vi "Autonomous Independent.vi"   [LabVIEW 2019]
doc: "This VI is called when autonomous begins, and will automatically be terminated when autonomous ends. You can carry out timed or sensor driven robot movement independently without needing to return to the caller."
uses:
  <vilib>/Rock Robotics/WPI/Utilities/WPI_GetSetVariantRefNum.vi
  <vilib>/Rock Robotics/Network Tables/NT Read String.vi
  <vilib>/Rock Robotics/Network Tables/NT Write Numeric Array.vi
  Robot Global Data.vi
panel:
  # "Be sure to right-click and choose Data Operations>>Make Current Value default if you want to save the array values with the VI"
types:
  T1 = typedef "WPI_JoystickDevRef.ctl" = cluster{"Device":T2}
  T2 = typedef "WPI_JoystickDeviceEnum.ctl" = enum16{"USB 0", "USB 1", "USB 2", "USB 3", "USB 4", "USB 5"}
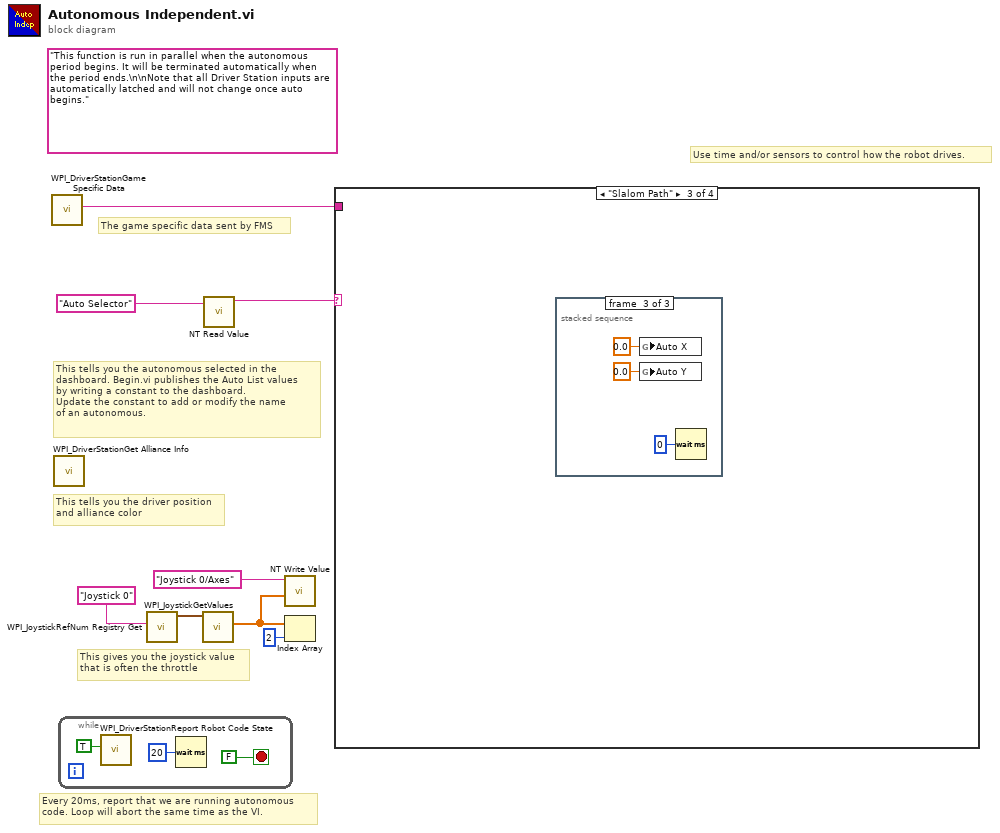
[diagram p0: block diagram]
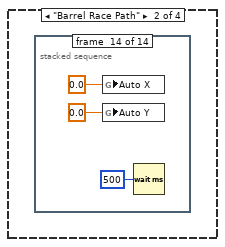
[diagram p3: hidden frame]
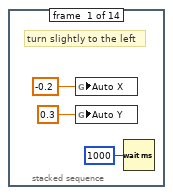
[diagram p4: hidden frame]
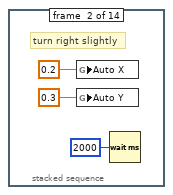
[diagram p5: hidden frame]
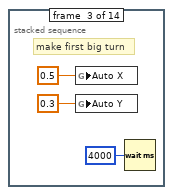
[diagram p6: hidden frame]
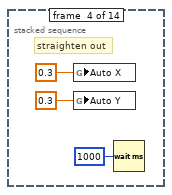
[diagram p7: hidden frame]
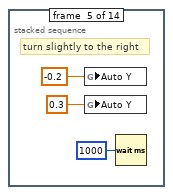
[diagram p8: hidden frame]
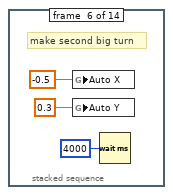
[diagram p9: hidden frame]
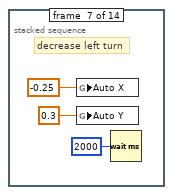
[diagram p10: hidden frame]
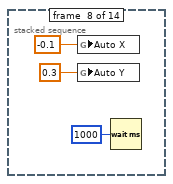
[diagram p11: hidden frame]
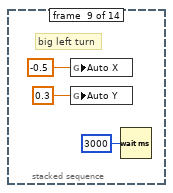
[diagram p12: hidden frame]
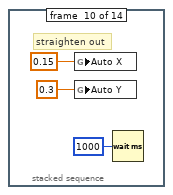
[diagram p13: hidden frame]
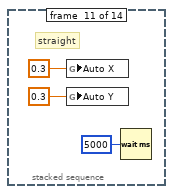
[diagram p14: hidden frame]
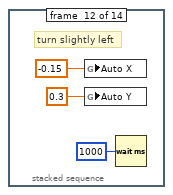
[diagram p15: hidden frame]
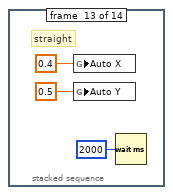
[diagram p16: hidden frame]
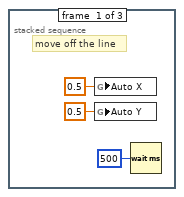
[diagram p17: hidden frame]
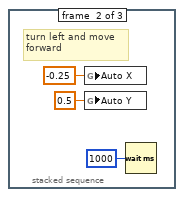
[diagram p18: hidden frame]
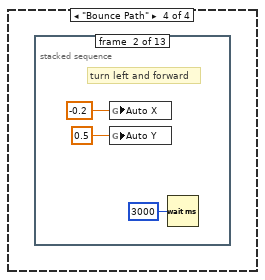
[diagram p19: hidden frame]
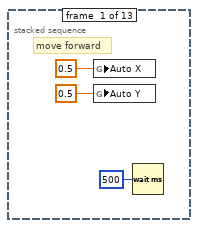
[diagram p20: hidden frame]
diagram:
  (unwired) "This function is run in parallel when the autonomous period begins. It will be terminated automatically when the period ends.\n\nNote that all Driver Station inputs are automatically latched and will not change once auto begins."
  # "The game specific data sent by FMS"
  # "This tells you the autonomous selected in the \ndashboard. Begin.vi publishes the Auto List values\nby writing a constant to the dashboard.\nUpdate the constant to add or modify the name\nof an autonomous."
  # "Every 20ms, report that we are running autonomous\ncode. Loop will abort the same time as the VI."
  # "This gives you the joystick value\nthat is often the throttle"
  # "Use time and/or sensors to control how the robot drives."
  # "This tells you the driver position\nand alliance color"
  n1 = call <vilib>:"WPI_DriverStationGame Specific Data.vi"() -> ("Game Specific Data"=w1:string)  [unwired: 11 in]
  n2 = call <vilib>:"WPI_DriverStationGet Alliance Info.vi"() -> ()  [unwired: 12 out]
  n3 = while {
    stop <- FALSE stop-if-true
    n4 = call <vilib>:"WPI_DriverStationReport Robot Code State.vi"("Autonomous"=TRUE) -> ()  [unwired: 10 in, 1 out]
    n5 = Wait (ms)(milliseconds to wait=u32 20) -> ()  [unwired: 1 out]
  }
  n6 = call <vilib>:"WPI_JoystickRefNum Registry Get.vi"("refnum name"="Joystick 0") -> ("JoystickDevRef"=w7:T1)  [unwired: 1 in, 9 out]
  n7 = call <vilib>:"WPI_JoystickGetValues.vi"("JoystickDevRef"=w7) -> ("Axes"=w3:dbl[])  [unwired: 6 in, 4 out]
  n8 = call-poly <vilib>:"NT Read Value.vi"("Name"="Auto Selector") -> ("String"=w4:string)  [unwired: 9 in, 1 out]
  n9 = call-poly <vilib>:"NT Write Value.vi"("Numeric Array"=w3, "Name"="Joystick 0/Axes") -> ()  [unwired: 9 in, 1 out]
  n10 = Index Array(array=w3, index=2) -> ()  [unwired: 1 out]
  n11 = case shown="\"Slalom Path\"" w4 {
    tunnel: w1 -> [_ _ _ _]
    frame Default {
      # "You can put your main auto here, or you can right-click on the case and make any\nother frame be the default case."
      # "This is the frame that will execute if no selection is made, or if it is not recognized"
    }
    frame "Barrel Race Path" {
      n12 = stacked-sequence {
        frame #0 {
          # "turn slightly to the left"
          n13 = global write "Robot Global Data.vi" "Auto X"(-0.2 ("Joystick X")) -> ()
          n14 = global write "Robot Global Data.vi" "Auto Y"(0.3 ("Joystick Y")) -> ()
          n15 = Wait (ms)(milliseconds to wait=u32 1000) -> ()  [unwired: 1 out]
        }
        frame #1 {
          # "turn right slightly"
          n16 = global write "Robot Global Data.vi" "Auto X"(0.2 ("Joystick X")) -> ()
          n17 = global write "Robot Global Data.vi" "Auto Y"(0.3 ("Joystick Y")) -> ()
          n18 = Wait (ms)(milliseconds to wait=u32 2000) -> ()  [unwired: 1 out]
        }
        frame #2 {
          # "make first big turn"
          n19 = global write "Robot Global Data.vi" "Auto X"(0.5 ("Joystick X")) -> ()
          n20 = global write "Robot Global Data.vi" "Auto Y"(0.3 ("Joystick Y")) -> ()
          n21 = Wait (ms)(milliseconds to wait=u32 4000) -> ()  [unwired: 1 out]
        }
        frame #3 {
          # "straighten out"
          n22 = global write "Robot Global Data.vi" "Auto X"(0.3 ("Joystick X")) -> ()
          n23 = global write "Robot Global Data.vi" "Auto Y"(0.3 ("Joystick Y")) -> ()
          n24 = Wait (ms)(milliseconds to wait=u32 1000) -> ()  [unwired: 1 out]
        }
        frame #4 {
          # "turn slightly to the right"
          n25 = global write "Robot Global Data.vi" "Auto Y"(-0.2 ("Joystick X")) -> ()
          n26 = global write "Robot Global Data.vi" "Auto Y"(0.3 ("Joystick Y")) -> ()
          n27 = Wait (ms)(milliseconds to wait=u32 1000) -> ()  [unwired: 1 out]
        }
        frame #5 {
          # "make second big turn"
          n28 = global write "Robot Global Data.vi" "Auto X"(-0.5 ("Joystick X")) -> ()
          n29 = global write "Robot Global Data.vi" "Auto Y"(0.3 ("Joystick Y")) -> ()
          n30 = Wait (ms)(milliseconds to wait=u32 4000) -> ()  [unwired: 1 out]
        }
        frame #6 {
          # "decrease left turn"
          n31 = global write "Robot Global Data.vi" "Auto X"(-0.25 ("Joystick X")) -> ()
          n32 = global write "Robot Global Data.vi" "Auto Y"(0.3 ("Joystick Y")) -> ()
          n33 = Wait (ms)(milliseconds to wait=u32 2000) -> ()  [unwired: 1 out]
        }
        frame #7 {
          n34 = global write "Robot Global Data.vi" "Auto X"(-0.1 ("Joystick X")) -> ()
          n35 = global write "Robot Global Data.vi" "Auto Y"(0.3 ("Joystick Y")) -> ()
          n36 = Wait (ms)(milliseconds to wait=u32 1000) -> ()  [unwired: 1 out]
        }
        frame #8 {
          # "big left turn"
          n37 = global write "Robot Global Data.vi" "Auto X"(-0.5 ("Joystick X")) -> ()
          n38 = global write "Robot Global Data.vi" "Auto Y"(0.3 ("Joystick Y")) -> ()
          n39 = Wait (ms)(milliseconds to wait=u32 3000) -> ()  [unwired: 1 out]
        }
        frame #9 {
          # "straighten out"
          n40 = global write "Robot Global Data.vi" "Auto X"(0.15 ("Joystick X")) -> ()
          n41 = global write "Robot Global Data.vi" "Auto Y"(0.3 ("Joystick Y")) -> ()
          n42 = Wait (ms)(milliseconds to wait=u32 1000) -> ()  [unwired: 1 out]
        }
        frame #10 {
          # "straight"
          n43 = global write "Robot Global Data.vi" "Auto X"(0.3 ("Joystick X")) -> ()
          n44 = global write "Robot Global Data.vi" "Auto Y"(0.3 ("Joystick Y")) -> ()
          n45 = Wait (ms)(milliseconds to wait=u32 5000) -> ()  [unwired: 1 out]
        }
        frame #11 {
          # "turn slightly left"
          n46 = global write "Robot Global Data.vi" "Auto X"(-0.15 ("Joystick X")) -> ()
          n47 = global write "Robot Global Data.vi" "Auto Y"(0.3 ("Joystick Y")) -> ()
          n48 = Wait (ms)(milliseconds to wait=u32 1000) -> ()  [unwired: 1 out]
        }
        frame #12 {
          # "straight"
          n49 = global write "Robot Global Data.vi" "Auto X"(0.4 ("Joystick X")) -> ()
          n50 = global write "Robot Global Data.vi" "Auto Y"(0.5 ("Joystick Y")) -> ()
          n51 = Wait (ms)(milliseconds to wait=u32 2000) -> ()  [unwired: 1 out]
        }
        frame #13 {
          n52 = global write "Robot Global Data.vi" "Auto X"(0.0 ("Joystick X")) -> ()
          n53 = global write "Robot Global Data.vi" "Auto Y"(0.0 ("Joystick Y")) -> ()
          n54 = Wait (ms)(milliseconds to wait=u32 500) -> ()  [unwired: 1 out]
        }
      }
    }
    frame "Slalom Path" {
      n55 = stacked-sequence {
        frame #0 {
          # "move off the line"
          n56 = global write "Robot Global Data.vi" "Auto X"(0.5 ("Auto X")) -> ()
          n57 = global write "Robot Global Data.vi" "Auto Y"(0.5 ("Auto Y")) -> ()
          n58 = Wait (ms)(milliseconds to wait=u32 500) -> ()  [unwired: 1 out]
        }
        frame #1 {
          # "turn left and move \nforward"
          n59 = global write "Robot Global Data.vi" "Auto X"(-0.25 ("Auto X")) -> ()
          n60 = global write "Robot Global Data.vi" "Auto Y"(0.5 ("Auto Y")) -> ()
          n61 = Wait (ms)(milliseconds to wait=u32 1000) -> ()  [unwired: 1 out]
        }
        frame #2 {
          n62 = global write "Robot Global Data.vi" "Auto X"(0.0 ("Auto X")) -> ()
          n63 = global write "Robot Global Data.vi" "Auto Y"(0.0 ("Auto Y")) -> ()
          n64 = Wait (ms)(milliseconds to wait=u32 0) -> ()  [unwired: 1 out]
        }
      }
    }
    frame "Bounce Path" {
      n65 = stacked-sequence {
        frame #0 {
          # "move forward"
          n66 = global write "Robot Global Data.vi" "Auto X"(0.5 ("Joystick X")) -> ()
          n67 = global write "Robot Global Data.vi" "Auto Y"(0.5 ("Joystick Y")) -> ()
          n68 = Wait (ms)(milliseconds to wait=u32 500) -> ()  [unwired: 1 out]
        }
        frame #1 {
          # "turn left and forward"
          n69 = global write "Robot Global Data.vi" "Auto X"(-0.2 ("Joystick X")) -> ()
          n70 = global write "Robot Global Data.vi" "Auto Y"(0.5 ("Joystick Y")) -> ()
          n71 = Wait (ms)(milliseconds to wait=u32 3000) -> ()  [unwired: 1 out]
        }
        frame #2 {
          # "turn right"
          n72 = global write "Robot Global Data.vi" "Auto X"(0.5 ("Joystick X")) -> ()
          n73 = global write "Robot Global Data.vi" "Auto Y"(0.25 ("Joystick Y")) -> ()
          n74 = Wait (ms)(milliseconds to wait=u32 3000) -> ()  [unwired: 1 out]
        }
        frame #3 {
          # "forward and left"
          n75 = global write "Robot Global Data.vi" "Auto X"(-0.2 ("Joystick X")) -> ()
          n76 = global write "Robot Global Data.vi" "Auto Y"(0.5 ("Joystick Y")) -> ()
          n77 = Wait (ms)(milliseconds to wait=u32 5000) -> ()  [unwired: 1 out]
        }
        frame #4 {
          # "U-turn"
          n78 = global write "Robot Global Data.vi" "Auto X"(-0.25 ("Joystick X")) -> ()
          n79 = global write "Robot Global Data.vi" "Auto Y"(0.5 ("Joystick Y")) -> ()
          n80 = Wait (ms)(milliseconds to wait=u32 3000) -> ()  [unwired: 1 out]
        }
        frame #5 {
          # "straight forward"
          n81 = global write "Robot Global Data.vi" "Auto X"(0.0 ("Joystick X")) -> ()
          n82 = global write "Robot Global Data.vi" "Auto Y"(0.5 ("Joystick Y")) -> ()
          n83 = Wait (ms)(milliseconds to wait=u32 3000) -> ()  [unwired: 1 out]
        }
        frame #6 {
          # "turn right"
          n84 = global write "Robot Global Data.vi" "Auto X"(0.5 ("Joystick X")) -> ()
          n85 = global write "Robot Global Data.vi" "Auto Y"(0.25 ("Joystick Y")) -> ()
          n86 = Wait (ms)(milliseconds to wait=u32 3000) -> ()  [unwired: 1 out]
        }
        frame #7 {
          # "straight forward"
          n87 = global write "Robot Global Data.vi" "Auto X"(0.5 ("Joystick X")) -> ()
          n88 = global write "Robot Global Data.vi" "Auto Y"(0.5 ("Joystick Y")) -> ()
          n89 = Wait (ms)(milliseconds to wait=u32 3000) -> ()  [unwired: 1 out]
        }
        frame #8 {
          # "left turn"
          n90 = global write "Robot Global Data.vi" "Auto X"(-0.5 ("Joystick X")) -> ()
          n91 = global write "Robot Global Data.vi" "Auto Y"(0.25 ("Joystick Y")) -> ()
          n92 = Wait (ms)(milliseconds to wait=u32 1500) -> ()  [unwired: 1 out]
        }
        frame #9 {
          # "straight forward"
          n93 = global write "Robot Global Data.vi" "Auto X"(0.5 ("Joystick X")) -> ()
          n94 = global write "Robot Global Data.vi" "Auto Y"(0.5 ("Joystick Y")) -> ()
          n95 = Wait (ms)(milliseconds to wait=u32 2000) -> ()  [unwired: 1 out]
        }
        frame #10 {
          # "turn left"
          n96 = global write "Robot Global Data.vi" "Auto X"(-0.25 ("Joystick X")) -> ()
          n97 = global write "Robot Global Data.vi" "Auto Y"(0.25 ("Joystick Y")) -> ()
          n98 = Wait (ms)(milliseconds to wait=u32 3000) -> ()  [unwired: 1 out]
        }
        frame #11 {
          # "slight left and forward"
          n99 = global write "Robot Global Data.vi" "Auto X"(-0.25 ("Joystick X")) -> ()
          n100 = global write "Robot Global Data.vi" "Auto Y"(0.5 ("Joystick Y")) -> ()
          n101 = Wait (ms)(milliseconds to wait=u32 5000) -> ()  [unwired: 1 out]
        }
        frame #12 {
          # "whip around and finish\nbackwards"
          n102 = global write "Robot Global Data.vi" "Auto X"(-0.25 ("Joystick X")) -> ()
          n103 = global write "Robot Global Data.vi" "Auto Y"(-0.5 ("Joystick Y")) -> ()
          n104 = Wait (ms)(milliseconds to wait=u32 3000) -> ()  [unwired: 1 out]
        }
      }
    }
  }
